vi "Call Load Bar_LV86.vi"   [LabVIEW 2009]
panel:
  # "This VI will make the front panel invisible while loading the subVI.\n\nThe subVI consists of an ActiveX control that is a loading bar.\n\nAfter loading is complete, the main VI will return to normal"
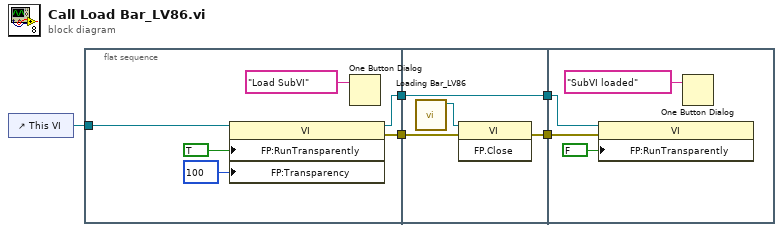
[diagram p0: block diagram]
diagram:
  n1 = control-ref of="This VI"() -> (w5:refnum<vi>)
  n2 = flat-sequence {
    tunnel: w5 -> [w10]
    tunnel: [w7] -> w3
    tunnel: [w6] -> w2
    tunnel: [w14] -> w4
    tunnel: w3 -> [w13]
    tunnel: w2 -> [w12]
    tunnel: [w12] -> w1
    tunnel: w4 -> [w17]
    tunnel: w1 -> [w16]
    frame #0 {
      n3 = property class="VI"(reference=w10, "FP:RunTransparently"=TRUE ("Front Panel Window:Run VI Transparently"), "FP:Transparency"=u8 100 ("Front Panel Window:Transparency")) -> (reference out=w6:refnum<vi>, error out=w7:errorcluster)  [unwired: 1 in]
      n4 = One Button Dialog(message="Load SubVI") -> ()  [unwired: 2 out]
    }
    frame #1 {
      n5 = call "Loading Bar_LV86.vi"() -> ("This VI"=w15:refnum<vi>)  [unwired: 11 out]
      n6 = invoke class="VI" method="FP.Close"(reference=w15, error in=w13) -> (error out=w14:errorcluster)  [unwired: 1 in, 2 out]
    }
    frame #2 {
      n7 = property class="VI"(reference=w16, error in=w17, "FP:RunTransparently"=FALSE ("Front Panel Window:Run VI Transparently")) -> ()  [unwired: 2 out]
      n8 = One Button Dialog(message="SubVI loaded") -> ()  [unwired: 2 out]
    }
  }
